vi "TestMenu.vi"() -> ()   [LabVIEW 2015, in "Menu.lvclass"]
uses:
  Menu.lvclass
panel:
  out "ItemTag 2":string
  out "ItemTag":string
  in  "stop":bool
  in  "Tree":string(tree)
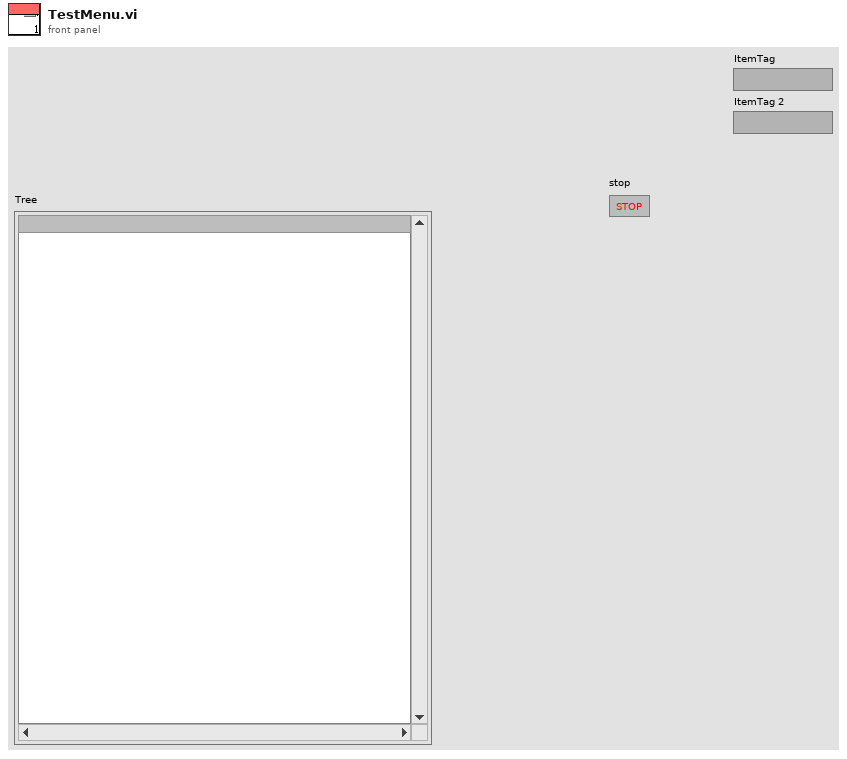
[diagram p1: front panel]
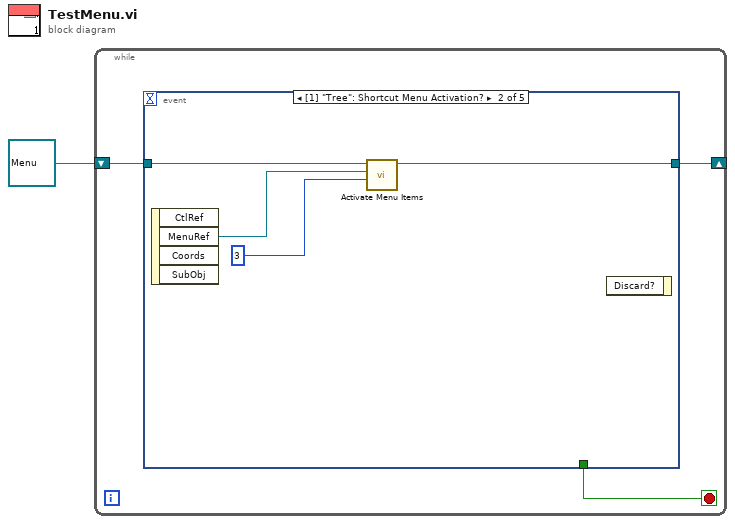
[diagram p0: block diagram]
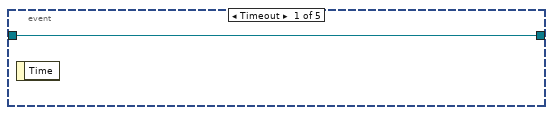
[diagram p2: hidden frame]
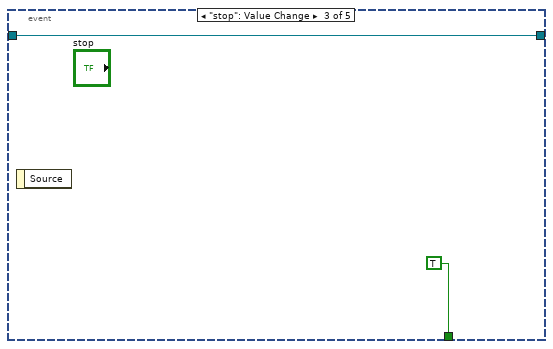
[diagram p3: hidden frame]
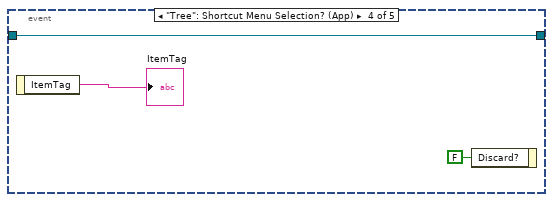
[diagram p4: hidden frame]
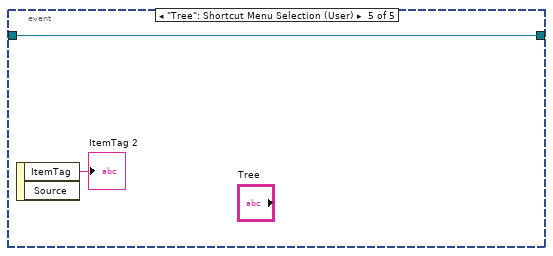
[diagram p5: hidden frame]
diagram:
  n1 = while {
    shift-right: [w2] -> _
    shift-left: refnum<class "Menu.lvclass"> refnum ("Menu.lvclass") -> [w4]
    stop <- w3 stop-if-true
    n2 = event shown="[1] \"Tree\": Shortcut Menu Activation?" {
      selector: _ -> [_ _ _ _ _]
      dyn-events: _ -> [_ _ _ _ _]
      timeout: _ -> [_ _ _ _ _]
      tunnel: w4 -> [w5 w9 w10 w14 w16]
      tunnel: [_ _ TRUE _ _] -> w3
      tunnel: [w5 w8 w10 w14 w16] -> w2
      event Timeout {
        n3 = event-data() -> ()  [unwired: 1 in, 1 out]
      }
      event "Tree": Shortcut Menu Activation? {
        n4 = event-data() -> ("MenuRef"=w7:refnum<k9>)  [unwired: 1 in, 3 out]
        n5 = call-dynamic "Activate Menu Items.vi"("State(0)"=3, "MenuRefnum"=w7, "Menu in"=w9) -> ("Menu out"=w8:refnum<class "Menu.lvclass">)  [unwired: 7 in, 1 out]
        n6 = event-data() -> ()  [unwired: 2 in, 1 out]
      }
      event "stop": Value Change {
        n7 = event-data() -> ()  [unwired: 1 in, 1 out]
      }
      event "Tree": Shortcut Menu Selection? (App) {
        n8 = event-data() -> ("ItemTag"=→"ItemTag":string)  [unwired: 1 in]
        n9 = event-data("Discard?"=FALSE) -> ()  [unwired: 1 in, 1 out]
      }
      event "Tree": Shortcut Menu Selection (User) {
        n10 = event-data() -> ("ItemTag"=→"ItemTag 2":string)  [unwired: 1 in, 1 out]
      }
    }
  }
